vi "DSF.Engine.Plugin.Rx.vi"(8 "error in (no error)":errorcluster, 10 "Transfer Group in":refnum<class "DSF.Engine.Transfer Group.lvclass">, 11 "UDP Plugin in":refnum<class "DSF.Plugin.UDP.lvclass">) -> (0 "error out":errorcluster, 2 "Transfer Group out":refnum<class "DSF.Engine.Transfer Group.lvclass">, 3 "UDP Plugin out":refnum<class "DSF.Plugin.UDP.lvclass">)   [LabVIEW 2017, in "DSF.Plugin.UDP.lvclass"]
uses:
  DSF.Plugin.UDP.lvclass
  Engine/Classes/Transfer/DSF.Engine.Transfer Group.lvclass
  Engine/Classes/Plugin/Plugin.lvclass
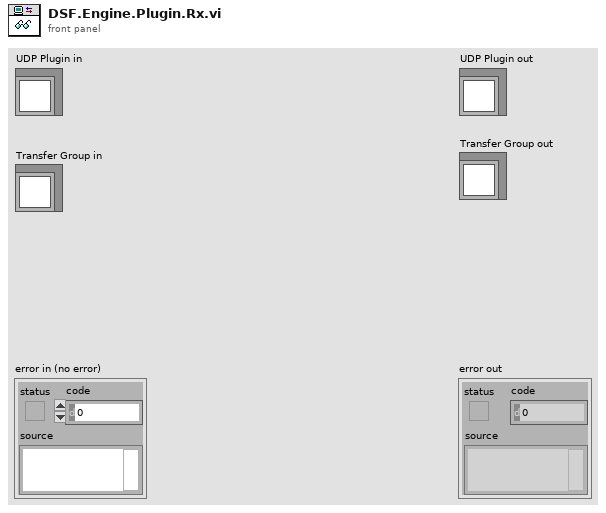
[diagram p1: front panel]
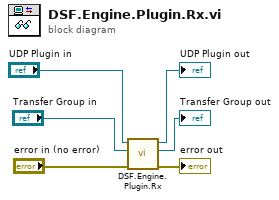
[diagram p0: block diagram]
diagram:
  n1 = call-parent "DSF.Engine.Plugin.Rx.vi"("error in (no error)"="error in (no error)", "Transfer Group in"="Transfer Group in", "Plugin in"="UDP Plugin in") -> ("error out"=→"error out":errorcluster, "Transfer Group out"=→"Transfer Group out":refnum<class "DSF.Engine.Transfer Group.lvclass">, "Plugin out"=→"UDP Plugin out":refnum<class "DSF.Plugin.UDP.lvclass">)  [unwired: 6 in]
